vi "HTTPMethod 1.vi"(7 "LabVIEW Web Service Request":refnum<class "Web Request.lvclass">, 8 "another_input":dbl, 11 "Some_input":string) -> (1 "Query":string, 3 "Some_output":string)   [LabVIEW 2015]
uses:
  <vilib>/wsapi/Web Request.lvclass
panel:
  # "Use the Web Service Request input terminal to call the VIs on the Web Services palette. Do not remove it from the connector pane unless you don't need access to the palette."
  # "Each additional control wired to the connector pane will be available as an input in the URL. To include an indicator in terminal-mode output (the default setting), it must also be wired to the connector pane."
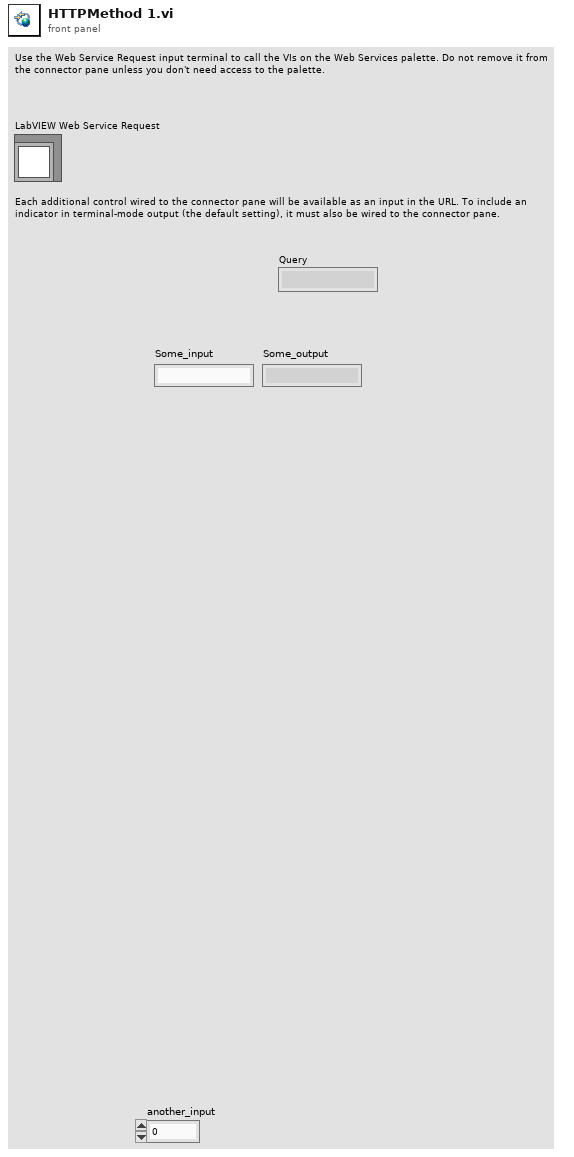
[diagram p1: front panel]
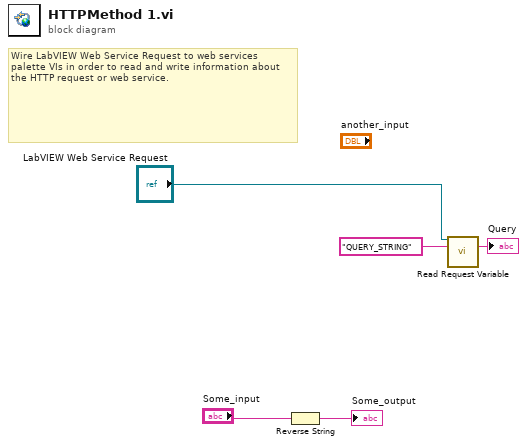
[diagram p0: block diagram]
diagram:
  # "Wire LabVIEW Web Service Request to web services palette VIs in order to read and write information about the HTTP request or web service."
  n1 = Reverse String(1:"Some_input") -> (0:→"Some_output":string)
  n2 = call <vilib>:"Read Request Variable.vi"("LabVIEW Web Service Request"="LabVIEW Web Service Request", "variable name"="QUERY_STRING") -> ("value"=→"Query":string)  [unwired: 11 in, 2 out]
